vi "Comunicacion serial.vi"(0 "VISA resource name":refnum<visa-resource-name>="COM1", 1 "baud rate":u32=9600, 2 "data bits":u16=8 min=5 max=8 step=1, 3 "parity":u16(ring) items=["None", "Odd", "Even", "Mark", "Space"], 4 "stop bits":u16(ring)=10 items=["1.0"=10, "1.5"=15, "2.0"=20], 7 "flow control":u16(ring) items=["None"=0, "XON/XOFF"=1, "RTS/CTS"=2, "DTR/DSR"=4]) -> ()   [LabVIEW 2010]
doc: "The Basic Serial Read and Write example performs a Serial Port Read, a Serial Port Write, or a combination of these actions. The user selects the actions (read or write) on the front panel. If both are selected, the VI will write the data first, read data, and then close the VISA session that is opened to the port. This VI will wait until the specified number of bytes is received at the port. Only the number of bytes specified will be read.\n\nINSTRUCTIONS:\n1) Select the serial resource and configuration parameters (baud rate, data bits, parity, stop bits, flow control).\n2) Select the operations to be performed. \n3) Connect the serial port to your device. If no device is available, perform a loopback test by doing one of the following. Short pins 2 and 3 on a RS-232 cable or short pin 4 to pin 8 and pin 5 to pin 9 on a RS-485/422 cable. \n4) Run the VI to see the data read. (The \"read string\" will match the \"string to write\" if a loopback test was performed.)\n\nNote: The parameters set for the serial port must match the parameters of the connected instrument or device. In this example, the bytes to read parameter specifies the number of bytes that the serial port reads. If there were more bytes at the port than the number specified in bytes to read, those bytes would not be read. Also, if you specify to read more bytes than the number of bytes actually read, you might receive a timeout error message.\n\nOn the block diagram, the Configure Serial Port VI sets the configuration parameters. The front panel displays the controls used to configure the basic parameters, such as baud rate, data bits, and parity. Constants configure the other parameters the user probably does not need set. After the VISA Configure Serial Port VI opens the VISA session and configures the port, the VI passes the VISA resource name to other VIs that perform operations on that VISA resource. The VISA Write function sends a command to the serial device and the VISA Read function returns data based on the command. The VISA Close function then closes the reference to the serial device. It is important to close the reference; otherwise communication through with that port through protocols other than VISA might not be possible."
uses:
  <vilib>/Instr/_visa.llb/VISA Configure Serial Port (Instr).vi
panel:
  in  "KP":dbl
  in  "Automatico":bool
  out "Ang.":dbl
  in  "Set Ang":dbl(slide) scale=55.0..90.0
  out "String":string
  in  "Velocidad":dbl(slide) scale=25.0..100.0
  out "Angulo":dynamicdata(graph)
  out "read buffer":string
  in  "stop":bool
  in  "delay before read (ms)":u32=500
  # "COM SERIAL"
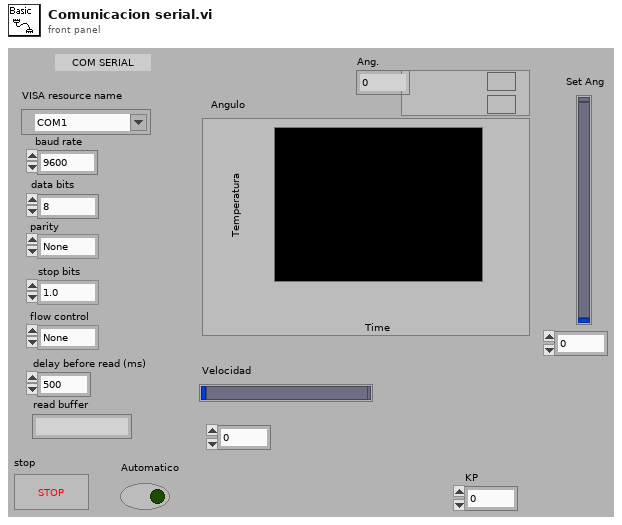
[diagram p1: front panel]
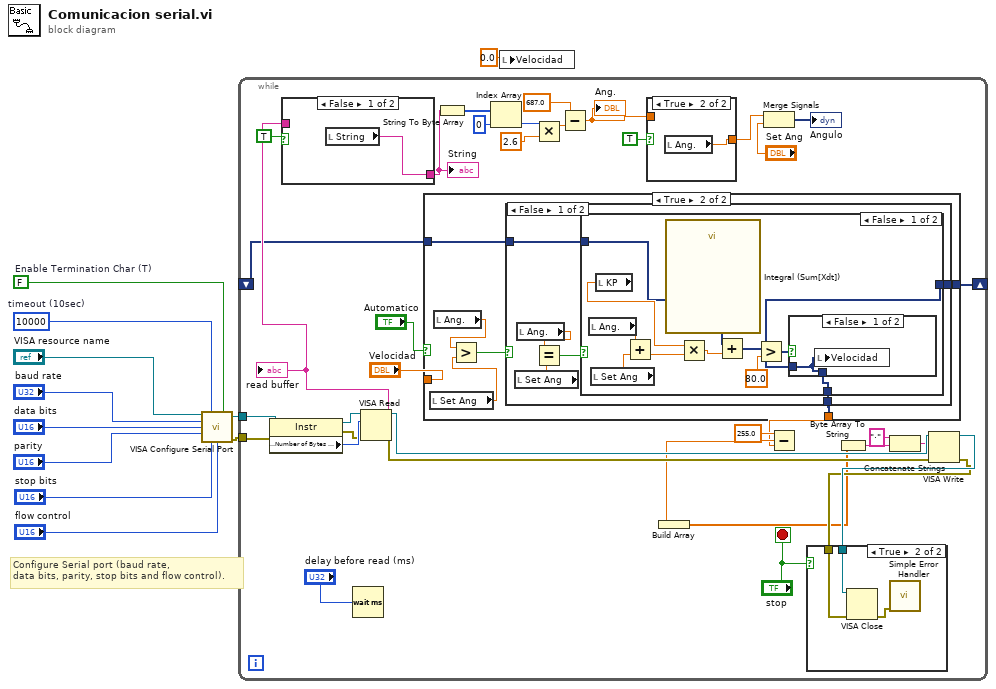
[diagram p0: block diagram]
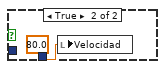
[diagram p4: hidden frame]
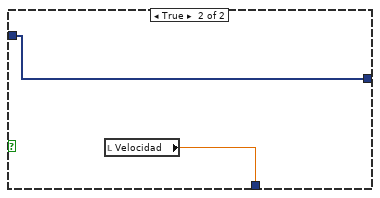
[diagram p5: hidden frame]
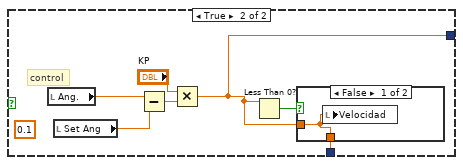
[diagram p6: hidden frame]
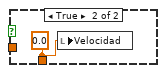
[diagram p7: hidden frame]
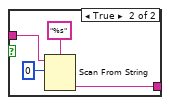
[diagram p8: hidden frame]
diagram:
  w6 = FALSE  # Enable Termination Char (T)
  w7 = u32 10000  # timeout (10sec)
  # "Configure Serial port (baud rate,\ndata bits, parity, stop bits and flow control)."
  n1 = call-poly "VISA Configure Serial Port"("VISA resource name"="VISA resource name", "timeout (10sec)"=w7, "Enable Termination\nChar (T)"=w6, "baud rate (9600)"="baud rate", "data bits (8)"="data bits", "parity (0:none)"="parity", "stop bits (10: 1 bit)"="stop bits", "flow control (0:none)"="flow control") -> ("VISA resource name out"=w9:refnum<visa-resource-name>, "error out"=w2:errorcluster)  [unwired: 6 in]
  n2 = while {
    tunnel: w2 -> [w46]
    tunnel: w9 -> [w42]
    shift-right: [w13] -> _
    shift-left: _ -> [w12]
    stop <- "stop" stop-if-true
    n3 = property class="Instr"(reference=w42, error in=w46) -> (reference out=w45:refnum<visa-resource-name>, error out=w43:errorcluster, "Serial Settings:Number of Bytes at Serial Port"=w44:u32)
    n4 = Wait (ms)(milliseconds to wait="delay before read (ms)") -> ()  [unwired: 1 out]
    n5 = VISA Read(VISA resource name=w45, byte count=w44, error in (no error)=w43) -> (VISA resource name out=w39:refnum<visa-resource-name>, read buffer=w35:string, error out=w38:errorcluster)  [unwired: 1 out]
    "read buffer" <- w35
    n6 = case shown="False" TRUE {
      tunnel: w35 -> [_ w89]
      tunnel: [w87 w88] -> w24
      frame False {
        n7 = local read "String"() -> (w87:string)
      }
      frame True {
        n8 = Scan From String(format string="%s", input string=w89, initial scan location=u32 0) -> (output 1=w88:string)  [unwired: 2 in, 3 out]
      }
    }
    "String" <- w24
    n9 = case shown="True" "Automatico" {
      tunnel: [w50 w53] -> w20
      tunnel: "Velocidad" -> [w50 _]
      tunnel: [_ w52] -> w13
      tunnel: w12 -> [_ w51]
      frame False {
      }
      frame True {
        n10 = local read "Set Ang"() -> (w55:dbl)
        n11 = local read "Ang."() -> (w56:dbl)
        n12 = Greater?(x=w56, y=w55) -> (0:w54:bool)
        n13 = case shown="False" w54 {
          tunnel: [w59 w82] -> w53
          tunnel: [w58 w78] -> w52
          tunnel: w51 -> [w57 _]
          frame False {
            n14 = local read "Set Ang"() -> (w61:dbl)
            n15 = local read "Ang."() -> (w62:dbl)
            n16 = Equal?(x=w62, y=w61) -> (x = y?=w60:bool)
            n17 = case shown="False" w60 {
              tunnel: [w70 w77] -> w59
              tunnel: [w65 w76] -> w58
              tunnel: w57 -> [w64 w76]
              frame False {
                n18 = local read "Ang."() -> (w73:dbl)
                n19 = local read "Set Ang"() -> (w69:dbl)
                n20 = local read "KP"() -> (w67:dbl)
                n21 = Add(x=w73, y=w69) -> (x+y=w68:dbl)
                n22 = call "Integral (Sum[Xdt])"("Signals"=w64) -> ("Result"=w63:dynamicdata)  [unwired: 5 in, 1 out]
                n23 = Multiply(x=w67, y=w68) -> (x*y=w66:dbl)
                n24 = Add(x=w63, y=w66) -> (x+y=w65:dynamicdata)
                n25 = Greater?(x=w65, y=80.0) -> (0:w72:dynamicdata)
                n26 = case shown="False" w72 {
                  tunnel: [w74 w75] -> w70
                  tunnel: w65 -> [w74 _]
                  frame False {
                    n27 = local write "Velocidad"(w74) -> ()
                  }
                  frame True {
                    w75 = 80.0 ("Velocidad")
                    n28 = local write "Velocidad"(w75) -> ()
                  }
                }
              }
              frame True {
                n29 = local read "Velocidad"() -> (w77:dbl)
              }
            }
          }
          frame True {
            (unwired) 0.1 ("Ajuste")
            # "control"
            n30 = local read "Ang."() -> (w84:dbl)
            n31 = local read "Set Ang"() -> (w79:dbl)
            n32 = Subtract(x=w84, y=w79) -> (x-y=w81:dbl)
            n33 = Multiply(x="KP", y=w81) -> (x*y=w78:dbl)
            n34 = Less Than 0?(x=w78) -> (x < 0?=w83:bool)
            n35 = case shown="False" w83 {
              tunnel: [w85 w86] -> w82
              tunnel: w78 -> [w85 _]
              frame False {
                n36 = local write "Velocidad"(w85) -> ()
              }
              frame True {
                w86 = 0.0 ("Velocidad")
                n37 = local write "Velocidad"(w86) -> ()
              }
            }
          }
        }
      }
    }
    n38 = String To Byte Array(string=w24) -> (unsigned byte array=w32:u8[])
    n39 = Index Array(array=w32, index=0) -> (element=w30:u8)
    n40 = Multiply(x=w30, y=2.6) -> (x*y=w19:dbl)
    n41 = Subtract(x=687.0 ("y"), y=w19) -> (x-y=w14:dbl)
    "Ang." <- w14
    n42 = case shown="True" TRUE {
      tunnel: [w48 w49] -> w16
      tunnel: w14 -> [w48 _]
      frame False {
      }
      frame True {
        n43 = local read "Ang."() -> (w49:dbl)
      }
    }
    n44 = Merge Signals(w16, "Set Ang") -> (→"Angulo":dynamicdata)
    n45 = Subtract(x=255.0 ("y"), y=w20) -> (x-y=w23:dbl)
    n46 = Build Array(w23) -> (w25:dbl[])
    n47 = Byte Array To String(unsigned byte array=w25) -> (string=w27:string)
    n48 = Concatenate Strings("·" ("string"), w27) -> (w28:string)
    n49 = VISA Write(VISA resource name=w39, write buffer=w28, error in (no error)=w38) -> (VISA resource name out=w37:refnum<visa-resource-name>, error out=w36:errorcluster)  [unwired: 1 out]
    n50 = case shown="True" "stop" {
      tunnel: w37 -> [_ w93]
      tunnel: w36 -> [_ w92]
      frame False {
      }
      frame True {
        n51 = VISA Close(VISA resource name=w93, error in (no error)=w92) -> (error out=w94:errorcluster)
        n52 = call <vilib>:"Simple Error Handler.vi"("error in (no error)"=w94) -> ()  [unwired: 4 in, 5 out]
      }
    }
  }
  n53 = local write "Velocidad"(0.0 ("Velocidad")) -> ()
